vi "Get Next Step.vi"(8 "error in (no error)":errorcluster, 11 "Output Sequencer in":refnum<class "Output Sequencer.lvclass">) -> (0 "error out":errorcluster, 1 "Next Cycle?":bool, 2 "Next Step":i32, 3 "Output Sequencer out":refnum<class "Output Sequencer.lvclass">, 5 "Sequencer State":T1)   [LabVIEW 2020, in "Output Sequencer.lvlib" / "Output Sequencer.lvclass"]
uses:
  Output Sequencer.lvclass
  Types/Sequencer State.ctl
  Output Sequencer.lvclass/Output Sequencer.ctl
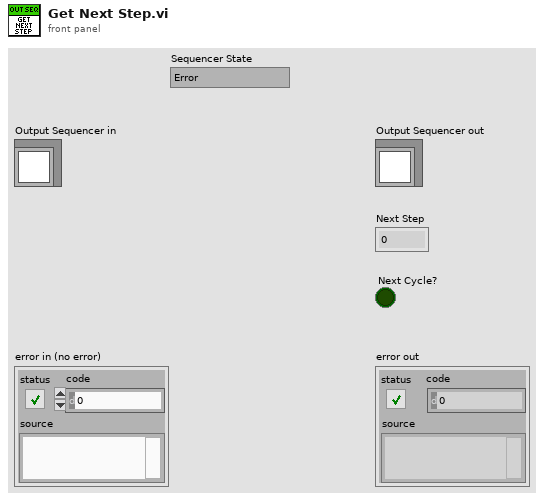
[diagram p1: front panel]
types:
  T1 = typedef "Output Sequencer.lvlib/Output Sequencer.lvclass/Sequencer State.ctl" = enum16{"Error", "Initialize", "Prepare channels", "Wait for test", "Wait for %.1f sec", "Wait for trigger", "Stop condition", "Wait for resume", "Running", "Paused", "No valid step", "Stopped"}
  T2 = typedef "Output Sequencer.lvlib/Output Sequencer.lvclass/Compiled Step.ctl" = cluster{"Precondition":T3, "Duration":dbl, "Mode":string, "Delay Between Values":dbl, "Analog Values":T3[], "Digital Values":T3[], "Postcondition":T3, "On True":string, "On False":string}
  T3 = typedef "Output Sequencer.lvlib/Output Sequencer.lvclass/Expression Data.ctl" = cluster{"Empty?":bool, "Expression":refnum<class "mupExpr.lvclass">, "Variable Names":string[]}
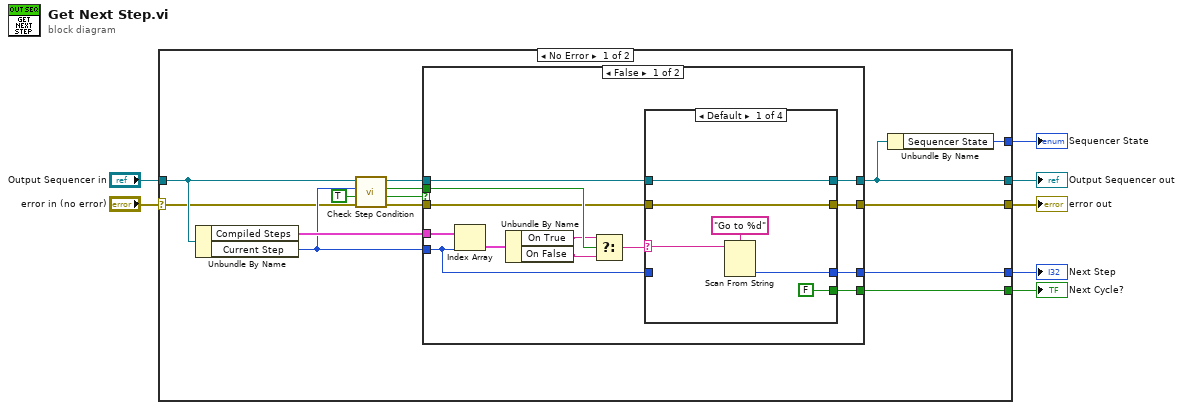
[diagram p0: block diagram]
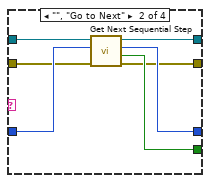
[diagram p2: hidden frame]
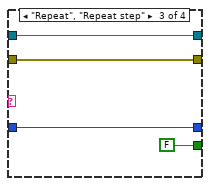
[diagram p3: hidden frame]
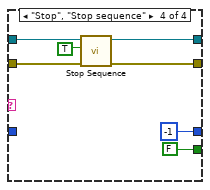
[diagram p4: hidden frame]
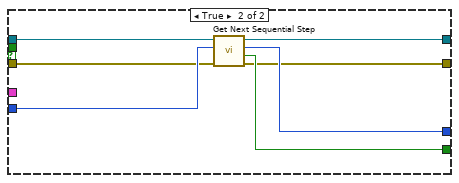
[diagram p5: hidden frame]
diagram:
  n1 = case shown="No Error" "error in (no error)" {
    selector: "error in (no error)" -> [w8 w66]
    tunnel: [w21 _] -> w7
    tunnel: [w20 _] -> w6
    tunnel: "Output Sequencer in" -> [w19 w67]
    tunnel: [w12 w66] -> w4
    tunnel: [w11 w67] -> w3
    tunnel: [w10 _] -> w2
    frame No Error {
      n2 = Unbundle By Name(w19) -> ("Compiled Steps"=w18:T2[], "Current Step"=w9:i32)
      n3 = call "Check Step Condition.vi"("error in (no error)"=w8, "Postcondition?"=TRUE, "Step Number"=w9, "Output Sequencer in"=w19) -> ("error out"=w13:errorcluster, "Check skipped"=w17:bool, "Condition passed"=w16:bool, "Output Sequencer out"=w14:refnum<class "Output Sequencer.lvclass">)  [unwired: 4 in]
      n4 = case shown="False" w17 {
        tunnel: w18 -> [w34 _]
        tunnel: w16 -> [w32 _]
        tunnel: w9 -> [w24 w65]
        tunnel: [w27 w63] -> w20
        tunnel: [w28 w62] -> w21
        tunnel: w14 -> [w26 w64]
        tunnel: [w25 w61] -> w11
        tunnel: w13 -> [w23 w60]
        tunnel: [w22 w59] -> w12
        frame False {
          n5 = Index Array(array=w34, index=w24) -> (element=w33:T2)
          n6 = Unbundle By Name(w33) -> ("On True"=w31:string, "On False"=w30:string)
          n7 = Select(t=w31, s=w32, f=w30) -> (s? t:f=w29:string)
          n8 = case shown="Default" w29 {
            selector: w29 -> [w37 _ _ _]
            tunnel: w24 -> [_ w47 w50 _]
            tunnel: [FALSE w45 FALSE ("Next Cycle?") FALSE] -> w28
            tunnel: [w36 w46 w50 -1] -> w27
            tunnel: w26 -> [w39 w44 w51 w56]
            tunnel: [w39 w43 w51 w55] -> w25
            tunnel: w23 -> [w35 w42 w48 w53]
            tunnel: [w35 w41 w48 w52] -> w22
            frame Default {
              n9 = Scan From String(format string="Go to %d", input string=w37) -> (output 1=w36:i32)  [unwired: 3 in, 3 out]
            }
            frame "", "Go to Next" {
              n10 = call "Get Next Sequential Step.vi"("error in (no error)"=w42, "Current Step"=w47, "Output Sequencer in"=w44) -> ("error out"=w41:errorcluster, "Next Cycle?"=w45:bool, "Next Step"=w46:i32, "Output Sequencer out"=w43:refnum<class "Output Sequencer.lvclass">)  [unwired: 4 in, 1 out]
            }
            frame "Repeat", "Repeat step" {
            }
            frame "Stop", "Stop sequence" {
              n11 = call "Stop Sequence.vi"("error in (no error)"=w53, "Use previous step values for Last values"=TRUE, "Output Sequencer in"=w56) -> ("error out"=w52:errorcluster, "Output Sequencer out"=w55:refnum<class "Output Sequencer.lvclass">)  [unwired: 6 in, 1 out]
            }
          }
        }
        frame True {
          n12 = call "Get Next Sequential Step.vi"("error in (no error)"=w60, "Current Step"=w65, "Output Sequencer in"=w64) -> ("error out"=w59:errorcluster, "Next Cycle?"=w62:bool, "Next Step"=w63:i32, "Output Sequencer out"=w61:refnum<class "Output Sequencer.lvclass">)  [unwired: 4 in, 1 out]
        }
      }
      n13 = Unbundle By Name(w11) -> ("Sequencer State"=w10:T1)
    }
    frame Error {
    }
  }
  "Next Cycle?" <- w7
  "Next Step" <- w6
  "Output Sequencer out" <- w3
  "error out" <- w4
  "Sequencer State" <- w2
